vi "R4CleanUp.vi"(8 "error in (no error)":errorcluster) -> (0 "error out":errorcluster)   [LabVIEW 2016]
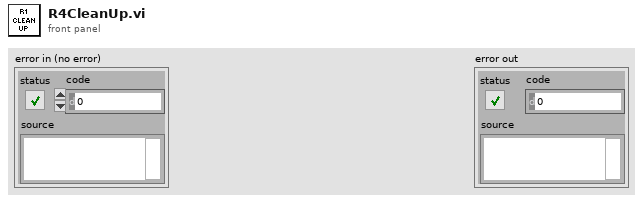
[diagram p1: front panel]
types:
  T1 = cluster{"Media Pump":bool, "Water Pump":bool, "Effluent Pump":bool, "Release Valve":bool, "Gas Pump":bool}
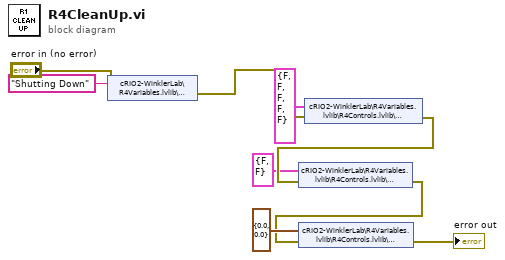
[diagram p0: block diagram]
diagram:
  n1 = shared-variable "cRIO2-WinklerLab\\R4Variables.lvlib\\R4Status"("Shutting Down" ("R1Status"), error in="error in (no error)") -> (error out=w7:errorcluster)
  n2 = shared-variable "cRIO2-WinklerLab\\R4Variables.lvlib\\R4Controls.lvlib\\R4SBRManual"(T1 {"Media Pump"=FALSE, "Water Pump"=FALSE, "Effluent Pump"=FALSE, "Release Valve"=FALSE, "Gas Pump"=FALSE} ("R4SBRManual"), error in=w7) -> (error out=w6:errorcluster)
  n3 = shared-variable "cRIO2-WinklerLab\\R4Variables.lvlib\\R4Controls.lvlib\\R4pHManual"(cluster{"Acid Pump":bool, "Base Pump":bool} {"Acid Pump"=FALSE, "Base Pump"=FALSE} ("R1pHManual"), error in=w6) -> (error out=w3:errorcluster)
  n4 = shared-variable "cRIO2-WinklerLab\\R4Variables.lvlib\\R4Controls.lvlib\\R4DOManual"(cluster{"Air MFC":dbl, "N2 MFC":dbl} {"Air MFC"=0.0, "N2 MFC"=0.0} ("R1DOManual"), error in=w3) -> (error out=→"error out":errorcluster)
